vi "ClusterwitharrayI16.vi"(1 "Cluster In":cluster{"Array In":i16[], "Numeric Input":i16}, 2 "Base":i16) -> (0 "Cluster Out":cluster{"Array Out":i16[], "Numeric Output":i16})   [LabVIEW 2010]
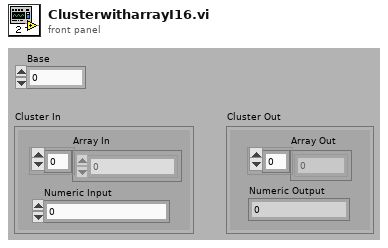
[diagram p1: front panel]
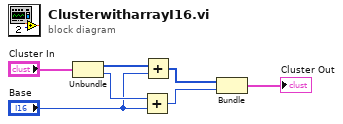
[diagram p0: block diagram]
diagram:
  n1 = Unbundle("Cluster In") -> ("Array In"=w7:i16[], "Numeric Input"=w6:i16)
  n2 = Add(x=w6, y="Base") -> (x+y=w4:i16)
  n3 = Add(x=w7, y="Base") -> (x+y=w5:i16[])
  n4 = Bundle(w5, w4) -> (→"Cluster Out":cluster{i16[], i16})  [unwired: 1 out]
